vi "Read configuration.vi"(8 "error in":errorcluster, 11 "State Machine editor node in":refnum<class "State Machine editor node.lvclass">) -> (0 "error out":errorcluster, 2 "configuration":refnum<class "NISE_CEF_serializable configuration.lvclass">, 3 "State Machine editor node out":refnum<class "State Machine editor node.lvclass">)   [LabVIEW 2021, in "State Machine editor node.lvclass"]
uses:
  State Machine editor node.lvclass
  <vilib>/NI/Configuration Framework/serializable configuration/NISE_CEF_serializable configuration.lvclass
  State Machine editor node.lvclass/State Machine editor node.ctl
  module/configuration/State Machine configuration.lvclass
  C:/Program Files (x86)/National Instruments/LabVIEW 2021/vi.lib/NI/Configuration Framework/serializable configuration/NISE_CEF_serializable configuration.lvclass
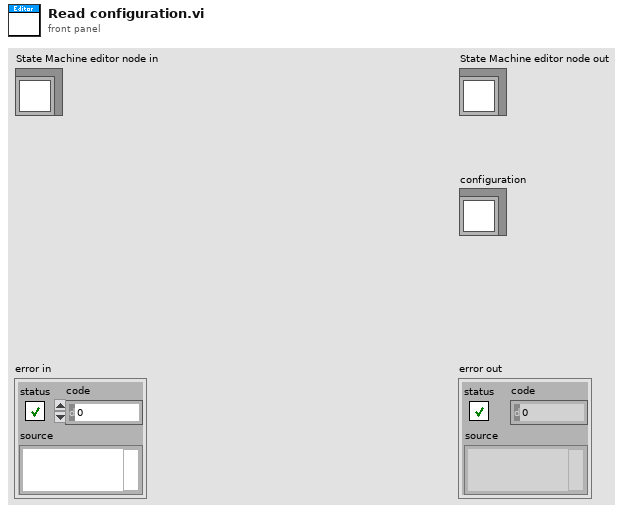
[diagram p1: front panel]
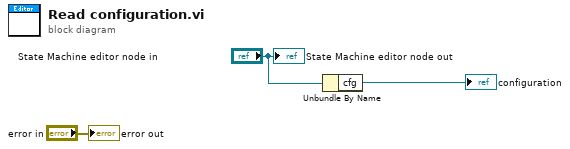
[diagram p0: block diagram]
diagram:
  n1 = Unbundle By Name("State Machine editor node in") -> ("cfg"=→"configuration":refnum<class "State Machine configuration.lvclass">)
  "error out" <- "error in"
  "State Machine editor node out" <- "State Machine editor node in"
